vi "Create I Chans_RTM.vi"(7 "Device Ref in":T1 format="%.0x", 8 "error in":errorcluster, 9 "Channels to Add":u16[](array[numeric]), 10 "Voltage Limit":dbl, 11 "Init Value":dbl) -> (0 "error out":errorcluster)   [LabVIEW 2018, in "NI PXI-4110 Programmable Power Supply Custom Device.lvlib"]
uses:
  NI PXI-4110 Programmable Power Supply Custom Device.lvlib
  <vilib>/NI Veristand/Custom Device API/Custom Device Item Ref.ctl
  <vilib>/NI Veristand/Custom Device API/Custom Device Channel.ctl
  <vilib>/NI Veristand/Custom Device API/Custom Device Channel Type.ctl
  4110_Global.vi
  <vilib>/NI Veristand/Custom Device API/Get Item Property (U16).vi
  <vilib>/NI Veristand/Custom Device API/Set Item Property (U16).vi
  <vilib>/NI VeriStand/Custom Device API/Custom Device API.lvlib
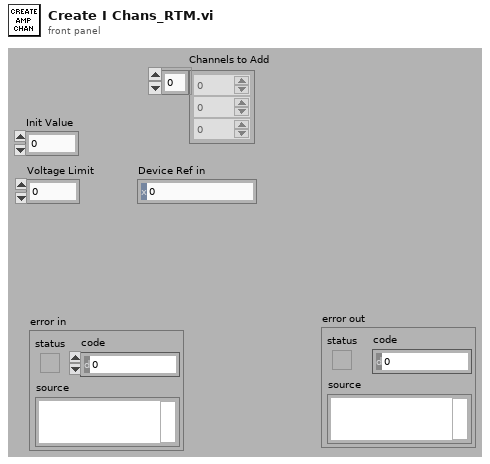
[diagram p1: front panel]
types:
  T1 = typedef "Custom Device API.lvlib/Custom Device Item Ref.ctl" = u64
  T2 = typedef "Custom Device API.lvlib/Custom Device Channel.ctl" = cluster{"Type":T3, "Units":string, "Default Value":dbl, "Faultable":bool, "Scalable":bool}
  T3 = typedef "Custom Device API.lvlib/Custom Device Channel Type.ctl" = enum16{"Input", "Output"}
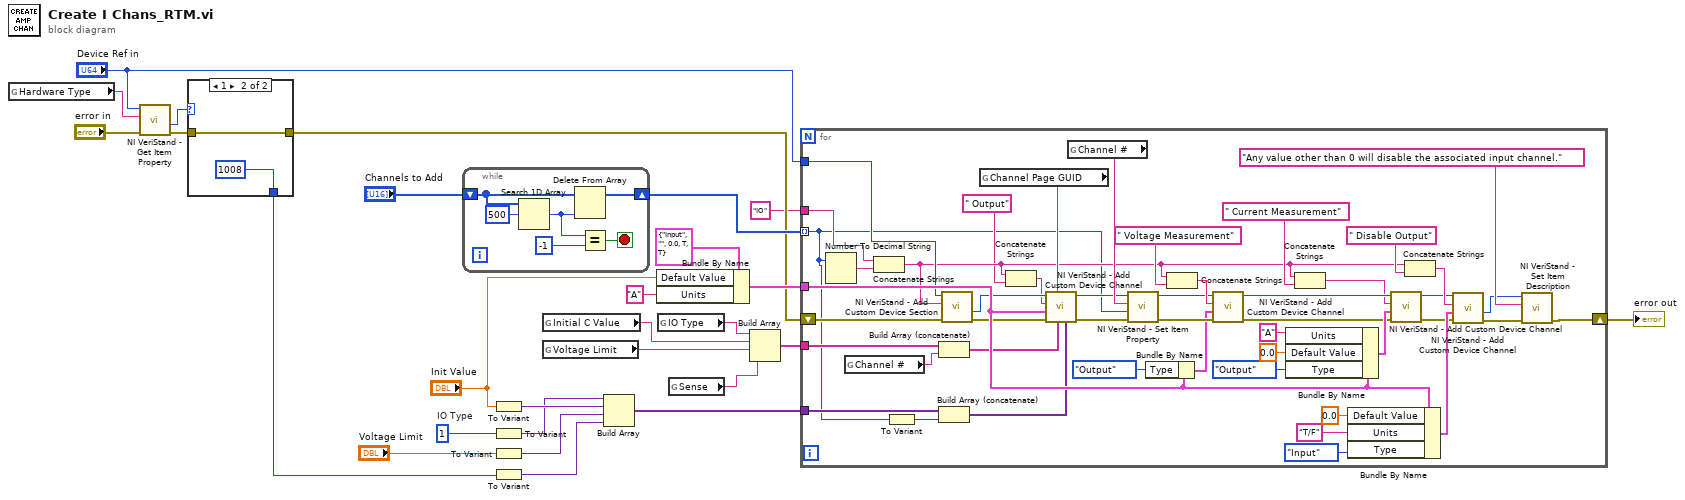
[diagram p0: block diagram]
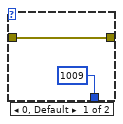
[diagram p2: hidden frame]
diagram:
  w16 = u16 1  # IO Type
  n1 = global read "4110_Global.vi" "Hardware Type"() -> (w9:string)
  n2 = call-poly <vilib>:"NI VeriStand - Get Item Property.vi"("error in (no error)"="error in", "Property Name"=w9, "Item Ref in"="Device Ref in") -> ("error out"=w6:errorcluster, "Value"=w7:u16)  [unwired: 5 in, 2 out]
  n3 = case shown="1" w7 {
    tunnel: w6 -> [w29 w31]
    tunnel: [w29 w31] -> w5
    tunnel: [1009 1008] -> w1
    frame 0, Default {
    }
    frame 1 {
    }
  }
  n4 = while {
    shift-right: [w33] -> w11
    shift-left: "Channels to Add" -> [w34]
    stop <- w32 stop-if-true
    n5 = Search 1D Array(1D array=w34, element=u16 500) -> (index of element=w36:i32)  [unwired: 1 in]
    n6 = Delete From Array(array=w34, index=w36) -> (array with subset deleted=w33:u16[])  [unwired: 1 in, 1 out]
    n7 = Equal?(x=w36, y=-1) -> (x = y?=w32:bool)
  }
  n8 = To Variant(anything="Init Value") -> (Variant=w24:variant)
  n9 = To Variant(anything=w16) -> (Variant=w23:variant)
  n10 = To Variant(anything="Voltage Limit") -> (Variant=w25:variant)
  n11 = To Variant(anything=w1) -> (Variant=w3:variant)
  n12 = global read "4110_Global.vi" "Initial C Value"() -> (w18:string)
  n13 = global read "4110_Global.vi" "Voltage Limit"() -> (w17:string)
  n14 = Build Array(w23, w24, w25, w3) -> (w26:variant[])
  n15 = Bundle By Name(cluster=T2 {"Type"=enum."Input", "Units"="", "Default Value"=0.0, "Faultable"=TRUE, "Scalable"=TRUE} ("Channel"), "Default Value"="Init Value", "Units"="A") -> (w20:T2)
  n16 = global read "4110_Global.vi" "IO Type"() -> (w19:string)
  n17 = global read "4110_Global.vi" "Sense"() -> (w4:string)
  n18 = Build Array(w19, w18, w17, w4) -> (w27:string[])
  n19 = for {
    shift-right: [w70] -> w22
    shift-left: w5 -> [w52]
    tunnel: w20 -> [w63]
    tunnel: "Device Ref in" -> [w51]
    tunnel: "IO" ("string") -> [w84]
    tunnel: w26 -> [w41]
    tunnel: w27 -> [w44]
    tunnel: w11 -> [w40] mode=indexing
    n20 = Number To Decimal String(number=w40) -> (decimal integer string=w83:string)  [unwired: 1 in]
    n21 = global read "4110_Global.vi" "Channel #"() -> (w43:string)
    n22 = Concatenate Strings(w84, w83) -> (w47:string)
    n23 = To Variant(anything=w40) -> (Variant=w39:variant)
    n24 = Build Array (concatenate)(w44, w43) -> (w42:string[])
    n25 = Build Array (concatenate)(w41, w39) -> (w38:variant[])
    n26 = call <vilib>:"NI VeriStand - Add Custom Device Section.vi"("error in (no error)"=w52, "Section Name"=w47, "Parent Ref in"=w51) -> ("error out"=w49:errorcluster, "Section Ptr"=w50:T1)  [unwired: 5 in, 2 out]
    n27 = global read "4110_Global.vi" "Channel Page GUID"() -> (w80:string)
    n28 = Concatenate Strings(w47, " Output") -> (w48:string)
    n29 = call <vilib>:"NI VeriStand - Add Custom Device Channel.vi"("Property Values"=w38, "Property names"=w42, "GUID (Default Channel)"=w80, "error in (no error)"=w49, "Channel"=w63, "Channel Name"=w48, "Parent Ref in"=w50) -> ("error out"=w82:errorcluster, "Parent Ref out"=w45:T1)  [unwired: 1 in, 2 out]
    n30 = global read "4110_Global.vi" "Channel #"() -> (w81:string)
    n31 = call-poly <vilib>:"NI VeriStand - Set Item Property.vi"("error in (no error)"=w82, "Value"=w40, "Property Name"=w81, "Item Ref in"=w45) -> ("error out"=w68:errorcluster, "Item Ref out"=w66:T1)  [unwired: 5 in, 1 out]
    n32 = Bundle By Name(cluster=w63, "Type"=Custom_Device_Channel_Type."Output") -> (w64:T2)
    n33 = Concatenate Strings(w47, " Voltage Measurement" ("string")) -> (w71:string)
    n34 = call <vilib>:"NI VeriStand - Add Custom Device Channel.vi"("error in (no error)"=w68, "Channel"=w64, "Channel Name"=w71, "Parent Ref in"=w66) -> ("error out"=w58:errorcluster, "Parent Ref out"=w57:T1)  [unwired: 4 in, 2 out]
    n35 = Bundle By Name(cluster=w63, "Units"="A", "Default Value"=0.0, "Type"=Custom_Device_Channel_Type."Output") -> (w62:T2)
    n36 = Concatenate Strings(w47, " Current Measurement" ("string")) -> (w53:string)
    n37 = Bundle By Name(cluster=w63, "Default Value"=0.0, "Units"="T/F", "Type"=Custom_Device_Channel_Type."Input") -> (w76:T2)
    n38 = call <vilib>:"NI VeriStand - Add Custom Device Channel.vi"("error in (no error)"=w58, "Channel"=w62, "Channel Name"=w53, "Parent Ref in"=w57) -> ("error out"=w55:errorcluster, "Parent Ref out"=w56:T1)  [unwired: 4 in, 2 out]
    n39 = Concatenate Strings(w47, " Disable Output" ("string")) -> (w73:string)
    n40 = call <vilib>:"NI VeriStand - Add Custom Device Channel.vi"("error in (no error)"=w55, "Channel"=w76, "Channel Name"=w73, "Parent Ref in"=w56) -> ("error out"=w77:errorcluster, "Channel Ref"=w78:T1)  [unwired: 4 in, 2 out]
    n41 = call <vilib>:"NI VeriStand - Set Item Description.vi"("error in (no error)"=w77, "Description"="Any value other than 0 will disable the associated input channel.", "Item Ref in"=w78) -> ("error out"=w70:errorcluster)  [unwired: 6 in, 2 out]
  }
  "error out" <- w22
